vi "weights_biases_export_sub.vi"(0 "format (%.3f)":string="%.3f", 1 "biases_1d":dbl[](array[numeric]), 2 "Export_biases_cvs":path=path "C:/Users/박원일/NEPL Dropbox/연구실 공용/뉴로모픽 과제/weights/biases_f_93.csv", 3 "weigths_2D":dbl[][](array[numeric]), 4 "Export_weights_cvs":path=path "C:/Users/박원일/NEPL Dropbox/연구실 공용/뉴로모픽 과제/weights/weights_f_93.csv") -> ()   [LabVIEW 2021]
uses:
  <vilib>/Utility/file.llb/Write Delimited Spreadsheet (DBL).vi
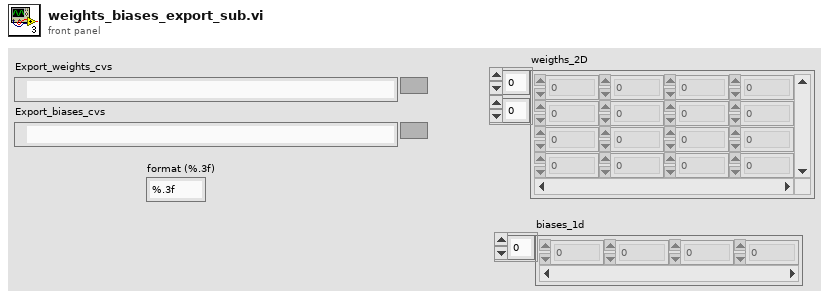
[diagram p1: front panel]
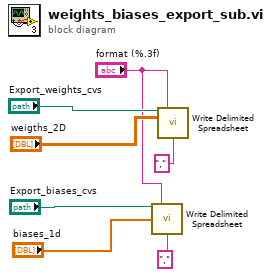
[diagram p0: block diagram]
diagram:
  n1 = call-poly <vilib>:"Write Delimited Spreadsheet.vi"("file path (dialog if empty)"="Export_biases_cvs", "format (%.3f)"="format (%.3f)", "1D data"="biases_1d", "delimiter (\\t)"="," ("delimiter (\\t)")) -> ()  [unwired: 10 in, 2 out]
  n2 = call-poly <vilib>:"Write Delimited Spreadsheet.vi"("file path (dialog if empty)"="Export_weights_cvs", "format (%.3f)"="format (%.3f)", "2D data"="weigths_2D", "delimiter (\\t)"="," ("delimiter (\\t)")) -> ()  [unwired: 10 in, 2 out]
